vi "Import Variable From String.vi"(8 "error in (no error)":errorcluster, 9 "section postfix":string, 10 "Configuration":string, 11 "CSM-Static-Variable-Manager in":refnum<class "CSM-Static-Variable-Manager.lvclass">) -> (0 "error out":errorcluster, 3 "CSM-Static-Variable-Manager out":refnum<class "CSM-Static-Variable-Manager.lvclass">)   [LabVIEW 2017, in "INI-Static-Variable-Support.lvlib" / "CSM-Static-Variable-Manager.lvclass"]
uses:
  CSM-Static-Variable-Manager.lvclass
  CSM-Static-Variable-Manager.lvclass/CSM-Static-Variable-Manager.ctl
  LabVIEW-Config/LabVIEW-Config.lvlib
  <userlib>/_NEVSTOP/Communicable State Machine(CSM)/addons/API-String-Arugments-Support/API String Arguments Support.lvlib
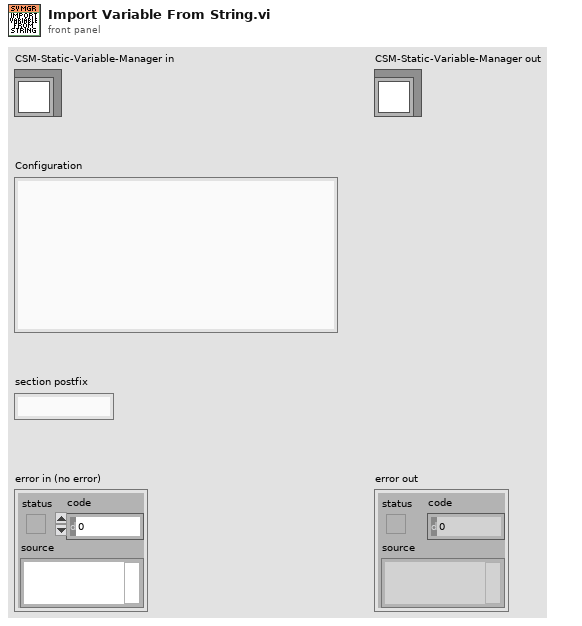
[diagram p1: front panel]
types:
  T1 = typedef "LabVIEW-Config.lvlib/Config.ctl" = cluster{"Path":path, "Lines":string[], "Tokens":T2[], "Modified?":bool}
  T2 = typedef "LabVIEW-Config.lvlib/LineToken.ctl" = enum8{"comment", "section", "key", "more"}
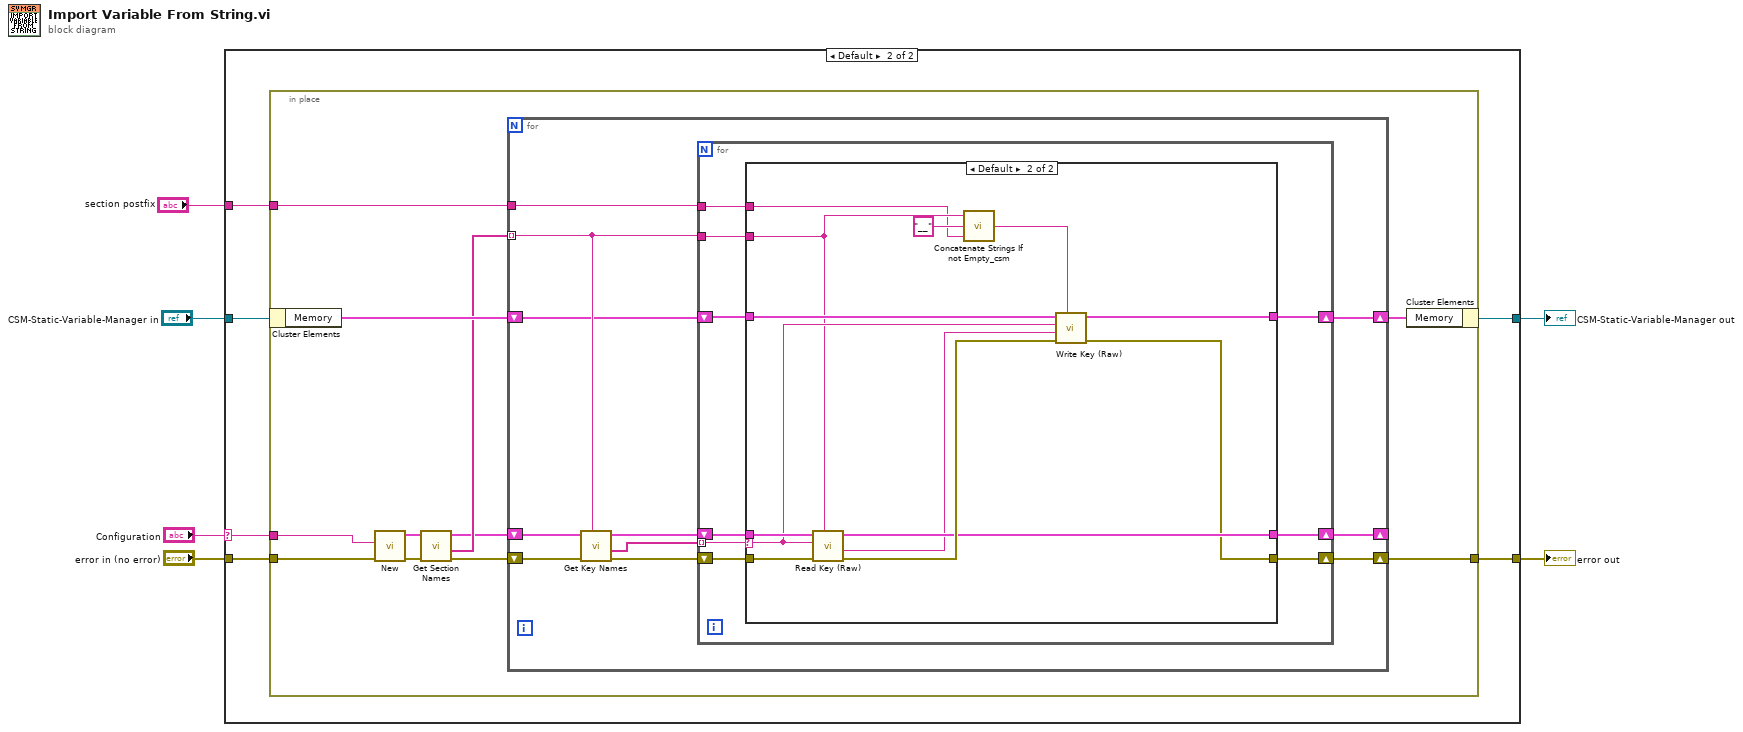
[diagram p0: block diagram]
diagram:
  n1 = case shown="Default" "Configuration" {
    selector: "Configuration" -> [_ w9]
    tunnel: [w7 w14] -> w4
    tunnel: "section postfix" -> [_ w13]
    tunnel: "CSM-Static-Variable-Manager in" -> [w8 w12]
    tunnel: [w8 w11] -> w2
    tunnel: "error in (no error)" -> [w7 w10]
    frame "" {
    }
    frame Default {
      n2 = in-place {
        in-place-border: [w22] -> w14
        in-place-border: w13 -> [w25]
        in-place-border: w10 -> [w17]
        in-place-border: w9 -> [w18]
        n3 = in-place-cluster #1(w12) -> ("Memory"=w24:T1)
        n4 = call "New.vi"("error in (no error)"=w17, "Text"=w18) -> ("error out"=w16:errorcluster, "Config"=w15:T1)  [unwired: 8 in]
        n5 = call "Get Section Names.vi"("error in (no error)"=w16, "Config in"=w15) -> ("error out"=w21:errorcluster, "Section Names"=w20:string[], "Config out"=w19:T1)  [unwired: 7 in]
        n6 = for {
          tunnel: w20 -> [w34] mode=indexing
          shift-right: [w32] -> w23
          shift-left: w24 -> [w33]
          shift-right: [w31] -> w22
          shift-left: w21 -> [w35]
          shift-right: [w30] -> _
          shift-left: w19 -> [w36]
          tunnel: w25 -> [w29]
          n7 = call "Get Key Names.vi"("Section Name"=w34, "error in (no error)"=w35, "Config in"=w36) -> ("error out"=w26:errorcluster, "Key Names"=w27:string[], "Config out"=w28:T1)  [unwired: 5 in, 1 out]
          n8 = for {
            tunnel: w34 -> [w38]
            tunnel: w27 -> [w39] mode=indexing
            shift-right: [w40] -> w31
            shift-left: w26 -> [w44]
            shift-right: [w43] -> w32
            shift-left: w33 -> [w42]
            shift-right: [w41] -> w30
            shift-left: w28 -> [w45]
            tunnel: w29 -> [w37]
            n9 = case shown="Default" w39 {
              selector: w39 -> [_ w53]
              tunnel: w45 -> [w47 w61]
              tunnel: w44 -> [w46 w60]
              tunnel: [w48 w59] -> w43
              tunnel: w42 -> [w48 w58]
              tunnel: [w47 w56] -> w41
              tunnel: [w46 w55] -> w40
              tunnel: w38 -> [_ w50]
              tunnel: w37 -> [_ w49]
              frame "Core.Current VI Reference" {
              }
              frame Default {
                n10 = call "Read Key (Raw).vi"("Section Name"=w50, "error in (no error)"=w60, "Key Name"=w53, "Config in"=w61) -> ("error out"=w57:errorcluster, "Content"=w54:string, "Config out"=w56:T1)  [unwired: 4 in, 1 out]
                n11 = call <userlib>:"Concatenate Strings If not Empty_csm.vi"("String"=w49, "seperator(:)"="__", "prefix"=w50) -> ("result"=w52:string)  [unwired: 2 in]
                n12 = call "Write Key (Raw).vi"("Section Name"=w52, "error in (no error)"=w57, "Content"=w54, "Key Name"=w53, "Config in"=w58) -> ("error out"=w55:errorcluster, "Config out"=w59:T1)  [unwired: 4 in, 1 out]
              }
            }
          }
        }
        n13 = in-place-cluster #1("Memory"=w23) -> (w11:refnum<class "CSM-Static-Variable-Manager.lvclass">)
      }
    }
  }
  "error out" <- w4
  "CSM-Static-Variable-Manager out" <- w2
